vi "FGVImageArray.vi"(7 "Enum":T1, 8 "error in":errorcluster) -> (0 "error out":errorcluster, 2 "ImageRefOut":refnum<data-value>[][](array[refnum]))   [LabVIEW 2016]
uses:
  controls/Enum.ctl
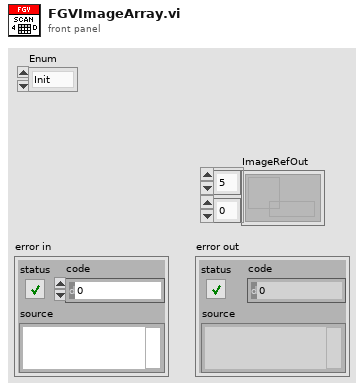
[diagram p1: front panel]
types:
  T1 = typedef "Enum.ctl" = enum16{"Init", "Read", "Write"}
  T2 = cluster{"channelsToSaveOut":u8[], "Units":string[], "Saving":cluster{"Fwd":i32[], "Bwd":i32[]}, "x":i32[]}
  T3 = cluster{"Width":dbl, "Height":dbl, "X Offset":dbl, "Y Offset":dbl, "Angle":dbl, "Pixels/Line":u16, "Lines":u16, "Time/Line":dbl, "Scan Rate":dbl}
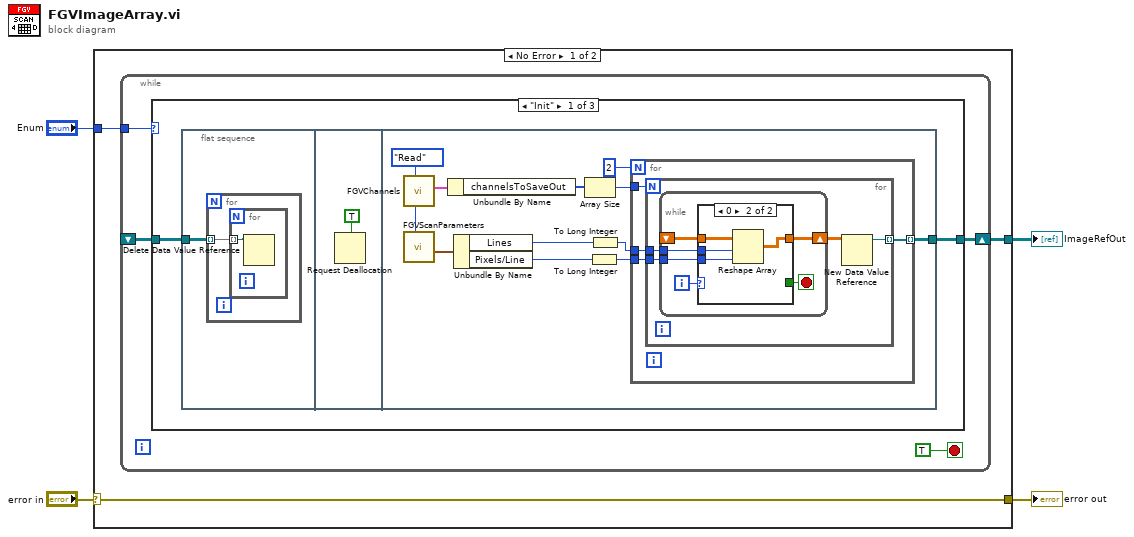
[diagram p0: block diagram]
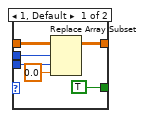
[diagram p2: hidden frame]
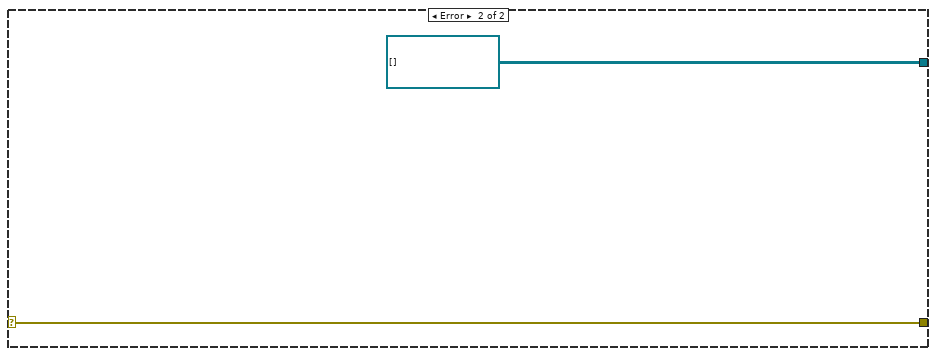
[diagram p5: hidden frame]
diagram:
  n1 = case shown="No Error" "error in" {
    selector: "error in" -> [w6 w56]
    tunnel: "Enum" -> [w7 _]
    tunnel: [w6 w56] -> w3
    tunnel: [w5 refnum<data-value>[][] []] -> w1
    frame No Error {
      n2 = while {
        tunnel: w7 -> [w10]
        shift-right: [w9] -> w5
        shift-left: _ -> [w8]
        stop <- TRUE stop-if-true
        n3 = case shown="\"Init\"" w10 {
          tunnel: [w13 w53 w54] -> w9
          tunnel: w8 -> [w12 w53 w54]
          frame "Init" {
            n4 = flat-sequence {
              tunnel: w12 -> [w14]
              tunnel: [w25] -> w13
              frame #0 {
                n5 = for {
                  tunnel: w14 -> [w15] mode=indexing
                  n6 = for {
                    tunnel: w15 -> [w16] mode=indexing
                    n7 = Delete Data Value Reference(data value reference=w16) -> ()  [unwired: 1 in, 2 out]
                  }
                }
              }
              frame #1 {
                n8 = Request Deallocation(TRUE ("flag")) -> ()
              }
              frame #2 {
                w22 = Enum."Read" ("Enum")
                n9 = call "FGVChannels.vi"("Enum"=w22) -> ("SavingChoiceOut"=w21:T2)  [unwired: 6 in, 4 out]
                n10 = call "FGVScanParameters.vi"("Enum"=w22) -> ("Scan Parameters Out"=w28:T3)  [unwired: 9 in, 1 out]
                n11 = Unbundle By Name(w21) -> ("channelsToSaveOut"=w20:u8[])
                n12 = Unbundle By Name(w28) -> ("Lines"=w27:u16, "Pixels/Line"=w26:u16)
                n13 = Array Size(array=w20) -> (size(s)=w19:i32)
                n14 = To Long Integer(number=w26) -> (32bit integer=w23:i32)
                n15 = To Long Integer(number=w27) -> (32bit integer=w24:i32)
                n16 = for {
                  N: 2 ("dimension size") -> [_]
                  tunnel: w24 -> [w32]
                  tunnel: w23 -> [w31]
                  tunnel: w19 -> [w30]
                  tunnel: [w29] -> w25 mode=indexing
                  n17 = for {
                    N: w30 -> [_]
                    tunnel: [w36] -> w29 mode=indexing
                    tunnel: w32 -> [w34]
                    tunnel: w31 -> [w35]
                    n18 = while {
                      shift-right: [w39] -> w33
                      shift-left: _ -> [w42]
                      tunnel: w35 -> [w40]
                      tunnel: w34 -> [w37]
                      i -> [w41]
                      stop <- w38 stop-if-true
                      n19 = case shown="0" w41 {
                        tunnel: w42 -> [w47 w49]
                        tunnel: [w46 w52] -> w39
                        tunnel: w37 -> [w45 w51]
                        tunnel: w40 -> [w44 w50]
                        tunnel: [TRUE _] -> w38
                        frame 1, Default {
                          n20 = Replace Array Subset(array=w47, new element=sgl 0.0, index (row)=w45, index (col)=w44) -> (w46:sgl[][])
                        }
                        frame 0 {
                          n21 = Reshape Array(w49, w51, w50) -> (w52:sgl[][])
                        }
                      }
                    }
                    n22 = New Data Value Reference(data value=w33) -> (data value reference=w36:refnum<data-value>)  [unwired: 1 in, 1 out]
                  }
                }
              }
            }
          }
          frame "Read", Default {
          }
          frame "Write" {
            # "If the terminal imageArray is not wired\n=> it is equal to its default value"
          }
        }
      }
    }
    frame Error {
    }
  }
  "error out" <- w3
  "ImageRefOut" <- w1
